vi "Autonomous Independent.vi"() -> ()   [LabVIEW 2023]
doc: "This VI is called when autonomous begins, and will automatically be terminated when autonomous ends. You can carry out timed or sensor driven robot movement independently without needing to return to the caller."
uses:
  <vilib>/Rock Robotics/WPI/ThirdParty/REV Robotics/REVLib/Typedef/Spark MAX Idle Mode.ctl
  <vilib>/Rock Robotics/WPI/SafetyOutput/WPI_SafetyOutputConfigMenu.ctl
  <vilib>/Rock Robotics/Network Tables/NT Read String.vi
  <vilib>/Rock Robotics/WPI/Utilities/WPI_GetSetVariantRefNum.vi
panel:
  out "Sensor Position 8":dbl
  out "Sensor Position 7":dbl
  out "?":dbl
  out "Sensor Position 6":dbl
  out "Sensor Position 5":dbl
  out "Sensor Position 4":dbl
  out "Sensor Position 3":dbl
  out "Sensor Position 2":dbl
  out "Sensor Position":dbl
  out "?":dbl
  # "Autonomous Independent.viBe sure to right-click and choose Data Operations>>Make Current Value default if you want to save the array values with the VI"
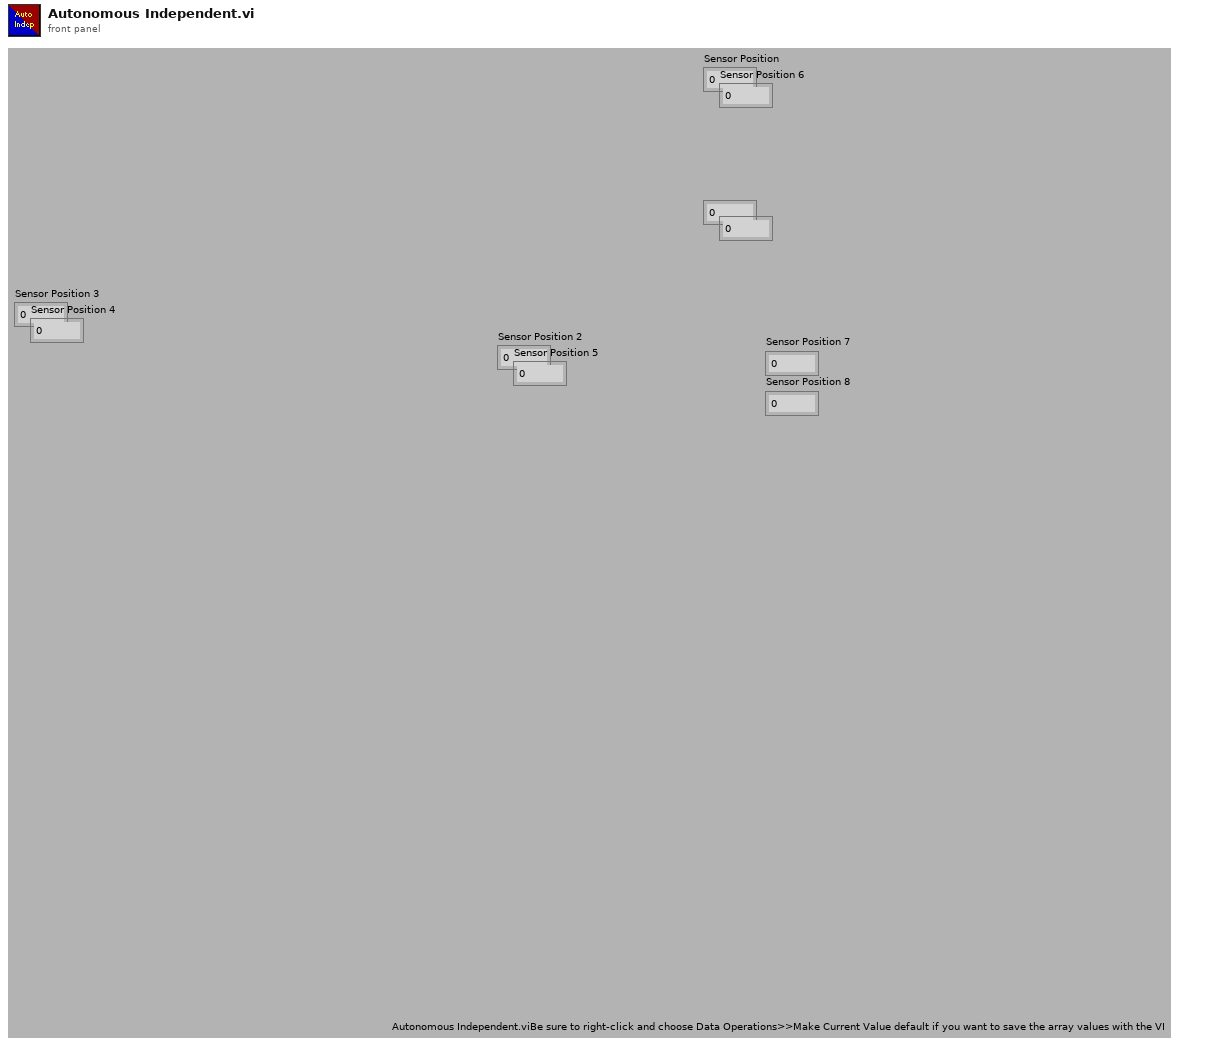
[diagram p1: front panel]
types:
  T1 = typedef "WPI_SafetyOutputConfigMenu.ctl" = enum16{"Enable", "Disable"}
  T2 = enum16{"ação 1", "ação 2", "ação 3", "ação 4", "ação 5", "ação 7", "ação 8"}
  T3 = typedef "Spark MAX Idle Mode.ctl" = enum16{"Coast", "Brake"}
  T4 = enum16{"ação 1", "ação 2", "ação 3", "ação 4", "ação 5"}
  T5 = typedef "WPI_RobotDriveDevRef.ctl" = cluster{"DevStatus":errorcluster, "Motors[]":T6[], "Square Inputs":bool, "Max Output":dbl}
  T6 = typedef "WPI_MotorControlDeviceRef.ctl" = cluster{"DeviceStatus":errorcluster, "Type":T7, "PWM":cluster{"PWM Channel":T8, "DeadBand":T9}, "CAN":cluster{"Device Number":u8, "SetOutput VI Ref":variant, "GetOutput VI Ref":variant, "Enable VI Ref":variant, "Disable VI Ref":variant, "Data":variant}, "Invert":bool, "DIO PWM":cluster{"PWM \"Enable\" Channel":T8, "DIOChannel":T10, "PWM Rate":dbl}}
  T7 = typedef "WPI_MotorControlType.ctl" = enum16{"PWM", "CAN", "DIO PWM"}
  T8 = typedef "FPGA_DIOPWMChannel.ctl" = enum8{"PWM 0", "PWM 1", "PWM 2", "PWM 3", "PWM 4", "PWM 5", "PWM 6", "PWM 7", "PWM 8", "PWM 9", "PWM MXP 0", "PWM MXP 1", "PWM MXP 2", "PWM MXP 3", "PWM MXP 4", "PWM MXP 5", "PWM MXP 6", "PWM MXP 7", "PWM MXP 8", "PWM MXP 9", "Invalid"}
  T9 = typedef "WPI_PWMDeadband.ctl" = cluster{"Name":string, "maxPositivePwm":i32, "minPositivePwm":i32, "centerPwm":i32, "maxNegativePwm":i32, "minNegativePwm":i32, "angularRange":u16}
  T10 = typedef "FPGA_DIOChannel.ctl" = enum8{"DIO 0", "DIO 1", "DIO 2", "DIO 3", "DIO 4", "DIO 5", "DIO 6", "DIO 7", "DIO 8", "DIO 9", "DIO MXP 0", "DIO MXP 1", "DIO MXP 2", "DIO MXP 3", "DIO MXP 4", "DIO MXP 5", "DIO MXP 6", "DIO MXP 7", "DIO MXP 8", "DIO MXP 9", "DIO MXP 10", "DIO MXP 11", "DIO MXP 12", "DIO MXP 13", "DIO MXP 14", "DIO MXP 15", "SPI Port CS1", "SPI Port CS2", "SPI Port CS3", "SPI Port MISO", "SPI Port MOSI", "Invalid"}
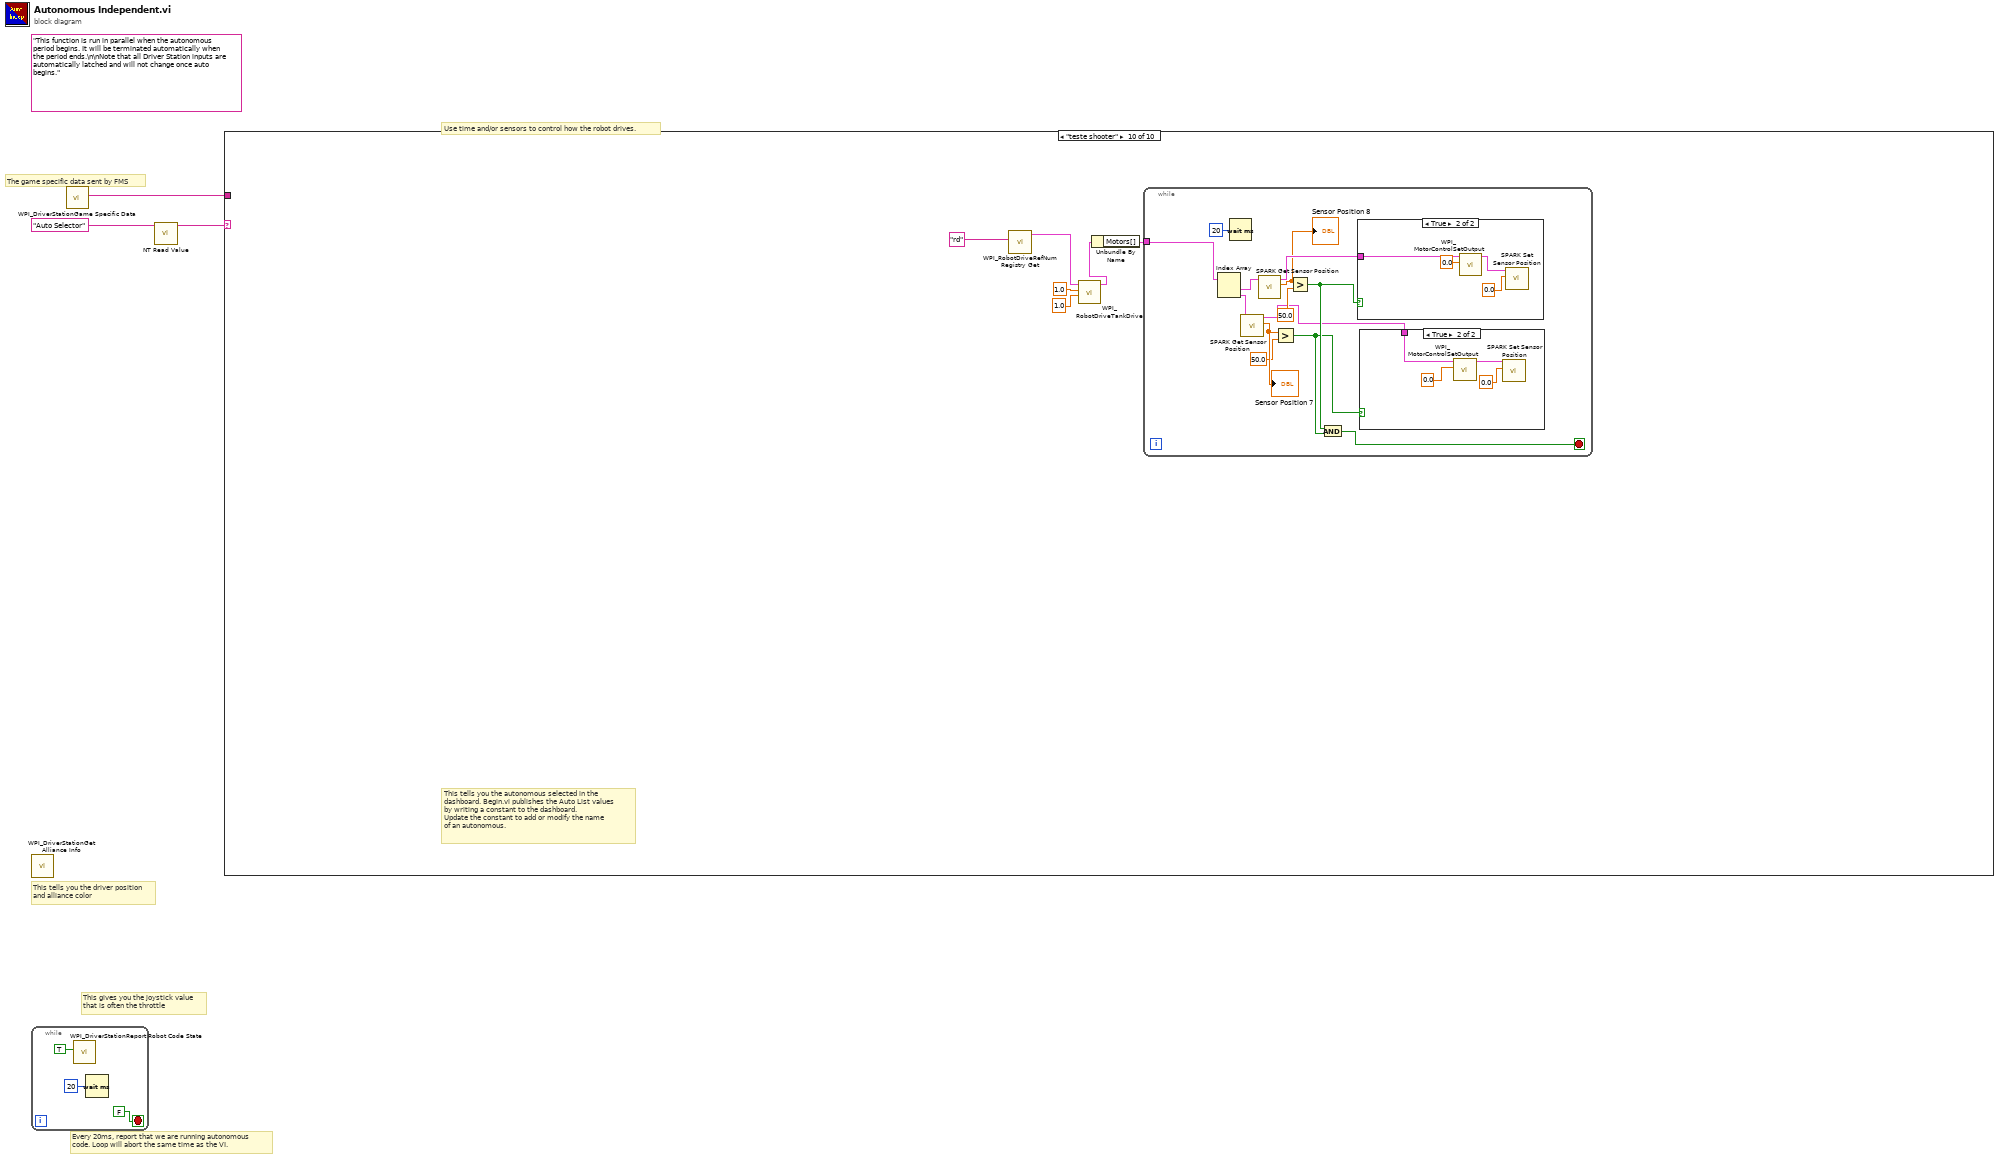
[diagram p0: block diagram]
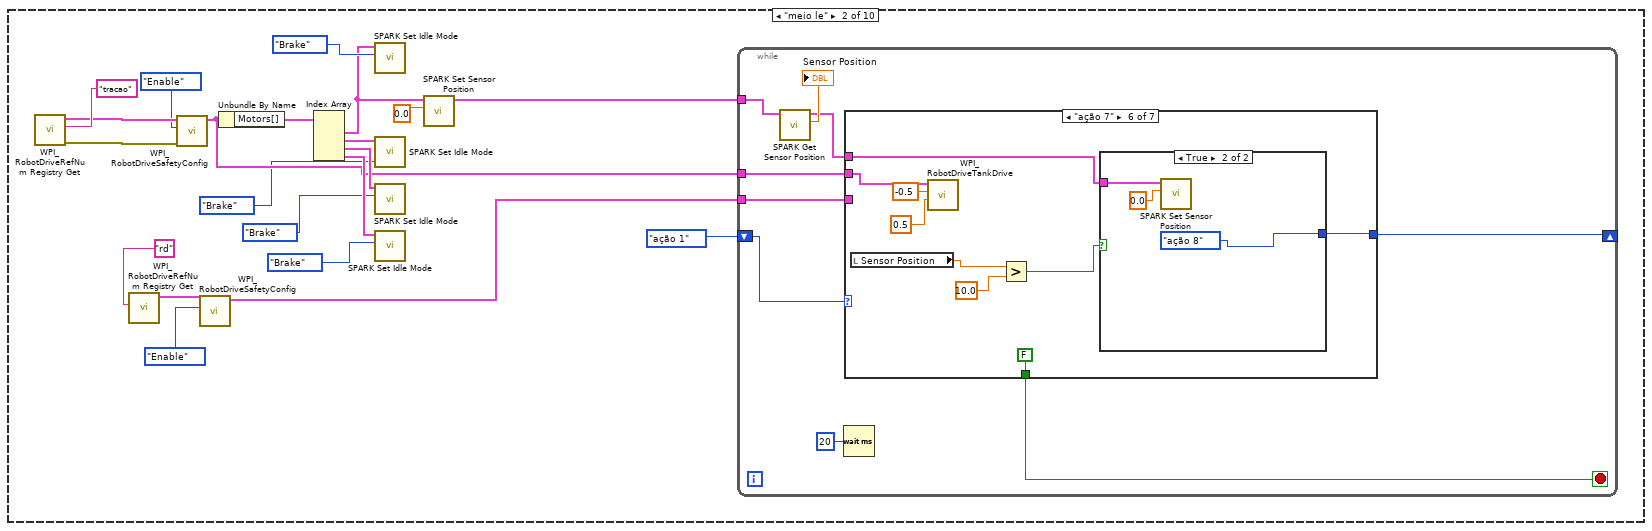
[diagram p3: hidden frame]
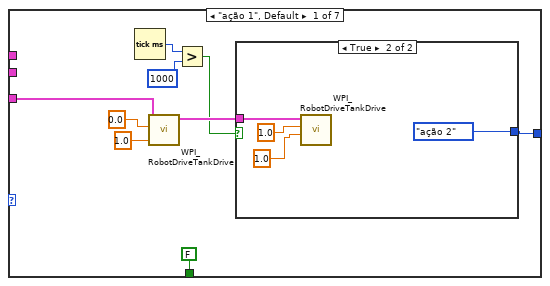
[diagram p4: hidden frame]
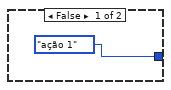
[diagram p5: hidden frame]
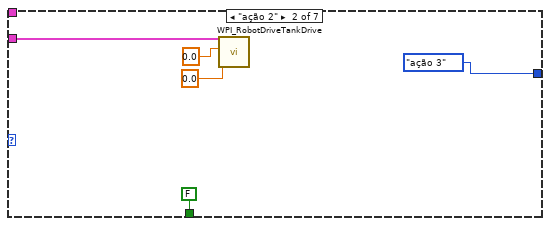
[diagram p6: hidden frame]
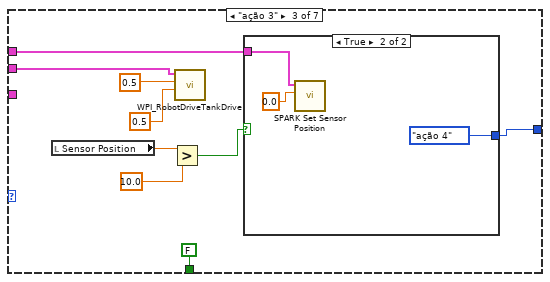
[diagram p7: hidden frame]
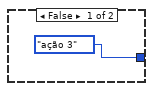
[diagram p8: hidden frame]
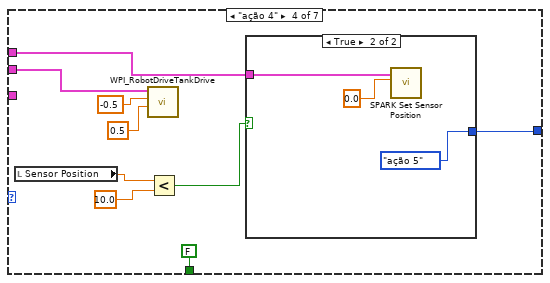
[diagram p9: hidden frame]
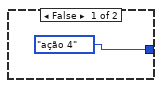
[diagram p10: hidden frame]
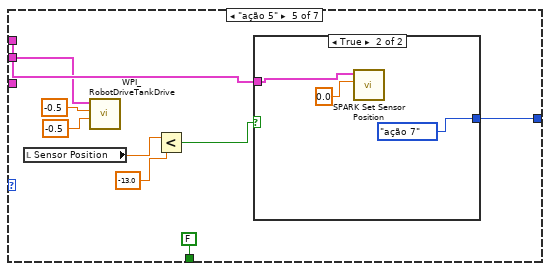
[diagram p11: hidden frame]
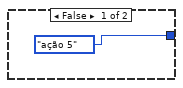
[diagram p12: hidden frame]
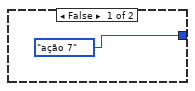
[diagram p13: hidden frame]
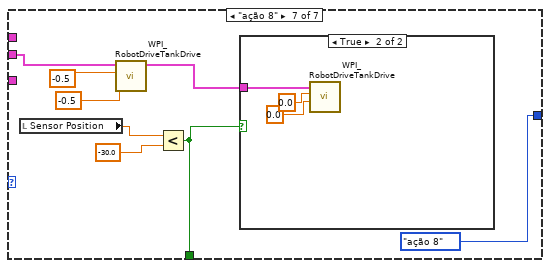
[diagram p14: hidden frame]
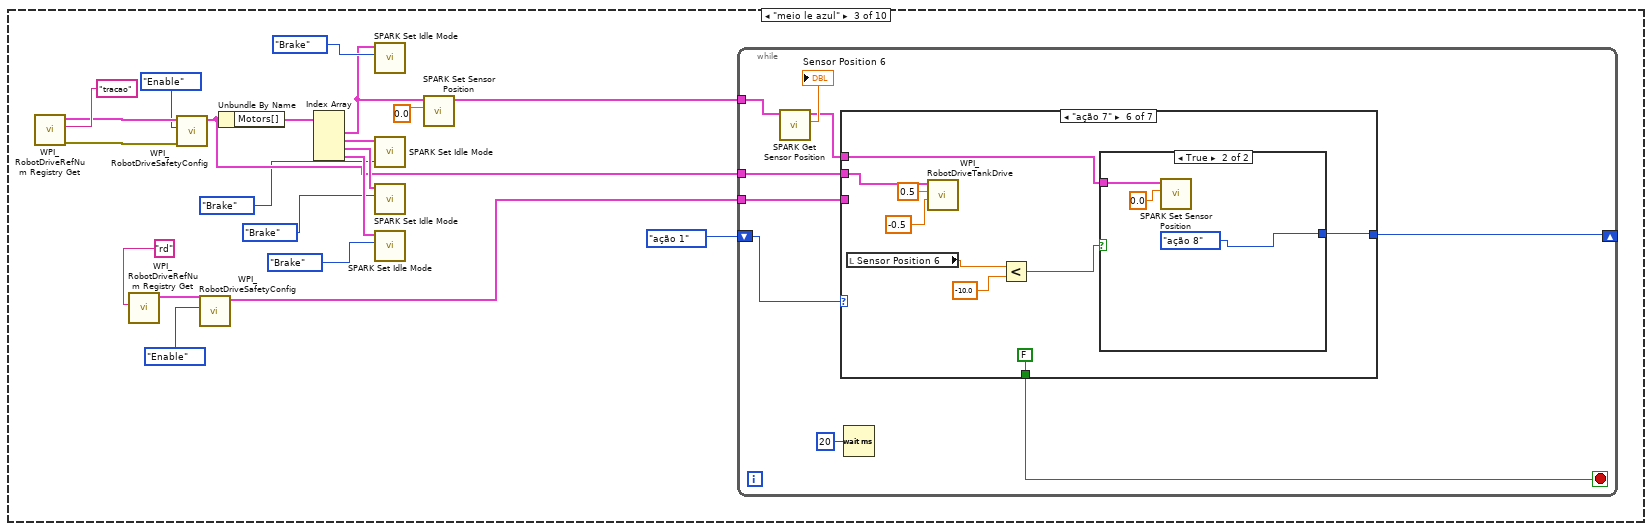
[diagram p16: hidden frame]
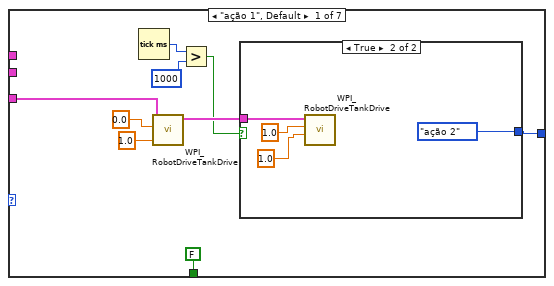
[diagram p17: hidden frame]
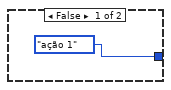
[diagram p18: hidden frame]
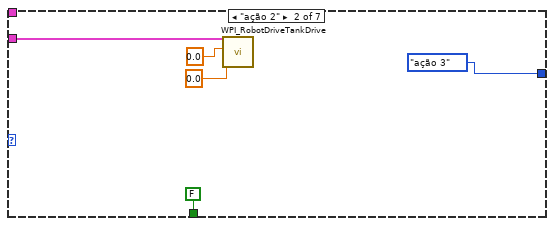
[diagram p19: hidden frame]
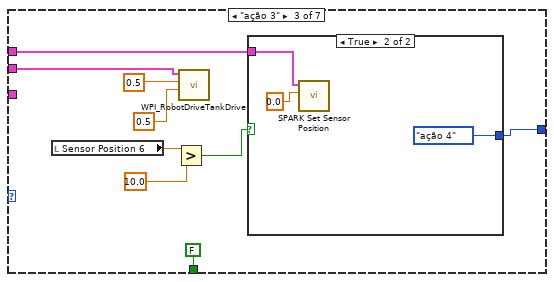
[diagram p20: hidden frame]
diagram:
  (unwired) "This function is run in parallel when the autonomous period begins. It will be terminated automatically when the period ends.\n\nNote that all Driver Station inputs are automatically latched and will not change once auto begins."
  # "The game specific data sent by FMS"
  # "This tells you the autonomous selected in the \ndashboard. Begin.vi publishes the Auto List values\nby writing a constant to the dashboard.\nUpdate the constant to add or modify the name\nof an autonomous."
  # "Every 20ms, report that we are running autonomous\ncode. Loop will abort the same time as the VI."
  # "This gives you the joystick value\nthat is often the throttle"
  # "Use time and/or sensors to control how the robot drives."
  # "This tells you the driver position\nand alliance color"
  n1 = call <vilib>:"WPI_DriverStationGet Alliance Info.vi"() -> ()  [unwired: 12 out]
  n2 = while {
    stop <- FALSE stop-if-true
    n3 = call <vilib>:"WPI_DriverStationReport Robot Code State.vi"("Autonomous"=TRUE) -> ()  [unwired: 10 in, 1 out]
    n4 = Wait (ms)(milliseconds to wait=u32 20) -> ()  [unwired: 1 out]
  }
  n5 = call <vilib>:"WPI_DriverStationGame Specific Data.vi"() -> ("Game Specific Data"=w1:string)  [unwired: 11 in]
  n6 = call-poly <vilib>:"NT Read Value.vi"("name"="Auto Selector" ("Name")) -> ("value"=w2:string)  [unwired: 8 in, 2 out]
  n7 = case shown="\"teste shooter\"" w2 {
    tunnel: w1 -> [_ _ _ _ _ _ _ _ _ _]
    frame Default {
    }
    frame "meio le" {
      n8 = call <vilib>:"WPI_RobotDriveRefNum Registry Get.vi"("refnum name"="tracao") -> ("error out"=w26:errorcluster, "RobotDriveDevRef"=w25:T5)  [unwired: 9 in]
      n9 = call <vilib>:"WPI_RobotDriveRefNum Registry Get.vi"("refnum name"="rd") -> ("RobotDriveDevRef"=w15:T5)  [unwired: 9 in, 1 out]
      n10 = call <vilib>:"WPI_RobotDriveSafetyConfig.vi"("error in (no error)"=w26, "mode"=WPI_SafetyOutputConfigMenu."Enable", "RobotDriveDevRef"=w25) -> ("RobotDriveDevRef"=w13:T5)  [unwired: 7 in, 1 out]
      n11 = call <vilib>:"WPI_RobotDriveSafetyConfig.vi"("mode"=WPI_SafetyOutputConfigMenu."Enable", "RobotDriveDevRef"=w15) -> ("RobotDriveDevRef"=w14:T5)  [unwired: 8 in, 1 out]
      n12 = Unbundle By Name(w13) -> ("Motors[]"=w24:T6[])
      n13 = Index Array(array=w24) -> (element #1=w17:T6, element #2=w21:T6, element #3=w20:T6, element #4=w19:T6)  [unwired: 4 in]
      n14 = call <vilib>:"SPARK Set Idle Mode.vi"("Idle Mode"=Spark_MAX_Idle_Mode."Brake", "MotorControlDeviceRef in"=w17) -> ()  [unwired: 8 in, 2 out]
      n15 = call <vilib>:"SPARK Set Idle Mode.vi"("Idle Mode"=Spark_MAX_Idle_Mode."Brake", "MotorControlDeviceRef in"=w21) -> ()  [unwired: 8 in, 2 out]
      n16 = call <vilib>:"SPARK Set Idle Mode.vi"("Idle Mode"=Spark_MAX_Idle_Mode."Brake", "MotorControlDeviceRef in"=w20) -> ()  [unwired: 8 in, 2 out]
      n17 = call <vilib>:"SPARK Set Idle Mode.vi"("Idle Mode"=Spark_MAX_Idle_Mode."Brake", "MotorControlDeviceRef in"=w19) -> ()  [unwired: 8 in, 2 out]
      n18 = call <vilib>:"SPARK Set Sensor Position.vi"("Position"=0.0, "MotorControlDeviceRef"=w17) -> ("MotorControlDeviceRef"=w12:T6)  [unwired: 8 in, 1 out]
      n19 = while {
        shift-right: [w33] -> _
        shift-left: T2."ação 1" -> [w35]
        tunnel: w14 -> [w34]
        tunnel: w13 -> [w32]
        tunnel: w12 -> [w30]
        stop <- w28 stop-if-true
        n20 = call <vilib>:"SPARK Get Sensor Position.vi"("MotorControlDevRef in"=w30) -> ("Sensor Position"=→"Sensor Position":dbl, "MotorControlDevRef out"=w29:T6)  [unwired: 7 in, 2 out]
        n21 = Wait (ms)(milliseconds to wait=u32 20) -> ()  [unwired: 1 out]
        n22 = case shown="\"ação 7\"" w35 {
          tunnel: w34 -> [w43 w55 _ _ _ _ _]
          tunnel: [w38 T2."ação 3" w57 w70 w83 w96 T2."ação 8"] -> w33
          tunnel: w32 -> [_ _ w64 w77 w87 w103 w115]
          tunnel: w29 -> [_ _ w58 w71 w90 w97 _]
          tunnel: [FALSE FALSE FALSE FALSE FALSE FALSE w109] -> w28
          frame "ação 1", Default {
            n23 = Tick Count (ms)() -> (millisecond timer value=w41:u32)
            n24 = call <vilib>:"WPI_RobotDriveTankDrive.vi"("Right axis value"=1.0, "Left axis value"=0.0, "RobotDriveDevRef"=w43) -> ("RobotDriveDevRef"=w42:T5)  [unwired: 6 in, 2 out]
            n25 = Greater?(x=w41, y=u32 1000) -> (0:w39:bool)
            n26 = case shown="True" w39 {
              tunnel: w42 -> [_ w48]
              tunnel: [T2."ação 1" T2."ação 2"] -> w38
              frame False {
              }
              frame True {
                n27 = call <vilib>:"WPI_RobotDriveTankDrive.vi"("Right axis value"=1.0 ("Left axis value"), "Left axis value"=1.0 ("Right axis value"), "RobotDriveDevRef"=w48) -> ()  [unwired: 6 in, 3 out]
              }
            }
          }
          frame "ação 2" {
            n28 = call <vilib>:"WPI_RobotDriveTankDrive.vi"("Right axis value"=0.0, "Left axis value"=0.0, "RobotDriveDevRef"=w55) -> ()  [unwired: 6 in, 3 out]
          }
          frame "ação 3" {
            n29 = local read "Sensor Position"() -> (w60:dbl)
            n30 = Greater?(x=w60, y=10.0) -> (0:w61:bool)
            n31 = call <vilib>:"WPI_RobotDriveTankDrive.vi"("Right axis value"=0.5 ("Left axis value"), "Left axis value"=0.5, "RobotDriveDevRef"=w64) -> ()  [unwired: 6 in, 3 out]
            n32 = case shown="True" w61 {
              tunnel: w58 -> [_ w68]
              tunnel: [T2."ação 3" T2."ação 4"] -> w57
              frame False {
              }
              frame True {
                n33 = call <vilib>:"SPARK Set Sensor Position.vi"("Position"=0.0, "MotorControlDeviceRef"=w68) -> ()  [unwired: 8 in, 2 out]
              }
            }
          }
          frame "ação 4" {
            n34 = local read "Sensor Position"() -> (w74:dbl)
            n35 = call <vilib>:"WPI_RobotDriveTankDrive.vi"("Right axis value"=0.5 ("Left axis value"), "Left axis value"=-0.5, "RobotDriveDevRef"=w77) -> ()  [unwired: 6 in, 3 out]
            n36 = Less?(x=w74, y=10.0) -> (x < y?=w72:bool)
            n37 = case shown="True" w72 {
              tunnel: w71 -> [_ w81]
              tunnel: [T2."ação 4" T2."ação 5"] -> w70
              frame False {
              }
              frame True {
                n38 = call <vilib>:"SPARK Set Sensor Position.vi"("Position"=0.0, "MotorControlDeviceRef"=w81) -> ()  [unwired: 8 in, 2 out]
              }
            }
          }
          frame "ação 5" {
            n39 = local read "Sensor Position"() -> (w86:dbl)
            n40 = call <vilib>:"WPI_RobotDriveTankDrive.vi"("Right axis value"=-0.5 ("Left axis value"), "Left axis value"=-0.5, "RobotDriveDevRef"=w87) -> ()  [unwired: 6 in, 3 out]
            n41 = Less?(x=w86, y=-13.0) -> (x < y?=w84:bool)
            n42 = case shown="True" w84 {
              tunnel: w90 -> [_ w93]
              tunnel: [T2."ação 5" T2."ação 7"] -> w83
              frame False {
              }
              frame True {
                n43 = call <vilib>:"SPARK Set Sensor Position.vi"("Position"=0.0, "MotorControlDeviceRef"=w93) -> ()  [unwired: 8 in, 2 out]
              }
            }
          }
          frame "ação 7" {
            n44 = local read "Sensor Position"() -> (w100:dbl)
            n45 = call <vilib>:"WPI_RobotDriveTankDrive.vi"("Right axis value"=0.5 ("Left axis value"), "Left axis value"=-0.5, "RobotDriveDevRef"=w103) -> ()  [unwired: 6 in, 3 out]
            n46 = Greater?(x=w100, y=10.0) -> (0:w98:bool)
            n47 = case shown="True" w98 {
              tunnel: w97 -> [_ w107]
              tunnel: [T2."ação 7" T2."ação 8"] -> w96
              frame False {
              }
              frame True {
                n48 = call <vilib>:"SPARK Set Sensor Position.vi"("Position"=0.0, "MotorControlDeviceRef"=w107) -> ()  [unwired: 8 in, 2 out]
              }
            }
          }
          frame "ação 8" {
            n49 = local read "Sensor Position"() -> (w112:dbl)
            n50 = call <vilib>:"WPI_RobotDriveTankDrive.vi"("Right axis value"=-0.5 ("Left axis value"), "Left axis value"=-0.5, "RobotDriveDevRef"=w115) -> ("RobotDriveDevRef"=w110:T5)  [unwired: 6 in, 2 out]
            n51 = Less?(x=w112, y=-30.0) -> (x < y?=w109:bool)
            n52 = case shown="True" w109 {
              tunnel: w110 -> [_ w118]
              frame False {
              }
              frame True {
                n53 = call <vilib>:"WPI_RobotDriveTankDrive.vi"("Right axis value"=0.0 ("Left axis value"), "Left axis value"=0.0, "RobotDriveDevRef"=w118) -> ()  [unwired: 6 in, 3 out]
              }
            }
          }
        }
      }
    }
    frame "meio le azul" {
      n54 = call <vilib>:"WPI_RobotDriveRefNum Registry Get.vi"("refnum name"="tracao") -> ("error out"=w138:errorcluster, "RobotDriveDevRef"=w137:T5)  [unwired: 9 in]
      n55 = call <vilib>:"WPI_RobotDriveRefNum Registry Get.vi"("refnum name"="rd") -> ("RobotDriveDevRef"=w127:T5)  [unwired: 9 in, 1 out]
      n56 = call <vilib>:"WPI_RobotDriveSafetyConfig.vi"("error in (no error)"=w138, "mode"=WPI_SafetyOutputConfigMenu."Enable", "RobotDriveDevRef"=w137) -> ("RobotDriveDevRef"=w125:T5)  [unwired: 7 in, 1 out]
      n57 = call <vilib>:"WPI_RobotDriveSafetyConfig.vi"("mode"=WPI_SafetyOutputConfigMenu."Enable", "RobotDriveDevRef"=w127) -> ("RobotDriveDevRef"=w126:T5)  [unwired: 8 in, 1 out]
      n58 = Unbundle By Name(w125) -> ("Motors[]"=w136:T6[])
      n59 = Index Array(array=w136) -> (element #1=w129:T6, element #2=w133:T6, element #3=w132:T6, element #4=w131:T6)  [unwired: 4 in]
      n60 = call <vilib>:"SPARK Set Idle Mode.vi"("Idle Mode"=Spark_MAX_Idle_Mode."Brake", "MotorControlDeviceRef in"=w129) -> ()  [unwired: 8 in, 2 out]
      n61 = call <vilib>:"SPARK Set Idle Mode.vi"("Idle Mode"=Spark_MAX_Idle_Mode."Brake", "MotorControlDeviceRef in"=w133) -> ()  [unwired: 8 in, 2 out]
      n62 = call <vilib>:"SPARK Set Idle Mode.vi"("Idle Mode"=Spark_MAX_Idle_Mode."Brake", "MotorControlDeviceRef in"=w132) -> ()  [unwired: 8 in, 2 out]
      n63 = call <vilib>:"SPARK Set Idle Mode.vi"("Idle Mode"=Spark_MAX_Idle_Mode."Brake", "MotorControlDeviceRef in"=w131) -> ()  [unwired: 8 in, 2 out]
      n64 = call <vilib>:"SPARK Set Sensor Position.vi"("Position"=0.0, "MotorControlDeviceRef"=w129) -> ("MotorControlDeviceRef"=w124:T6)  [unwired: 8 in, 1 out]
      n65 = while {
        shift-right: [w145] -> _
        shift-left: T2."ação 1" -> [w147]
        tunnel: w126 -> [w146]
        tunnel: w125 -> [w144]
        tunnel: w124 -> [w142]
        stop <- w140 stop-if-true
        n66 = call <vilib>:"SPARK Get Sensor Position.vi"("MotorControlDevRef in"=w142) -> ("Sensor Position"=→"Sensor Position 6":dbl, "MotorControlDevRef out"=w141:T6)  [unwired: 7 in, 2 out]
        n67 = case shown="\"ação 7\"" w147 {
          tunnel: w146 -> [w155 w167 _ _ _ _ _]
          tunnel: [w150 T2."ação 3" w169 w182 w195 w208 T2."ação 8"] -> w145
          tunnel: w144 -> [_ _ w176 w189 w199 w215 w227]
          tunnel: w141 -> [_ _ w170 w183 w202 w209 _]
          tunnel: [FALSE FALSE FALSE FALSE FALSE FALSE w221] -> w140
          frame "ação 1", Default {
            n68 = Tick Count (ms)() -> (millisecond timer value=w153:u32)
            n69 = call <vilib>:"WPI_RobotDriveTankDrive.vi"("Right axis value"=1.0, "Left axis value"=0.0, "RobotDriveDevRef"=w155) -> ("RobotDriveDevRef"=w154:T5)  [unwired: 6 in, 2 out]
            n70 = Greater?(x=w153, y=u32 1000) -> (0:w151:bool)
            n71 = case shown="True" w151 {
              tunnel: w154 -> [_ w160]
              tunnel: [T2."ação 1" T2."ação 2"] -> w150
              frame False {
              }
              frame True {
                n72 = call <vilib>:"WPI_RobotDriveTankDrive.vi"("Right axis value"=1.0 ("Left axis value"), "Left axis value"=1.0 ("Right axis value"), "RobotDriveDevRef"=w160) -> ()  [unwired: 6 in, 3 out]
              }
            }
          }
          frame "ação 2" {
            n73 = call <vilib>:"WPI_RobotDriveTankDrive.vi"("Right axis value"=0.0, "Left axis value"=0.0, "RobotDriveDevRef"=w167) -> ()  [unwired: 6 in, 3 out]
          }
          frame "ação 3" {
            n74 = local read "Sensor Position 6"() -> (w172:dbl)
            n75 = Greater?(x=w172, y=10.0) -> (0:w173:bool)
            n76 = call <vilib>:"WPI_RobotDriveTankDrive.vi"("Right axis value"=0.5 ("Left axis value"), "Left axis value"=0.5, "RobotDriveDevRef"=w176) -> ()  [unwired: 6 in, 3 out]
            n77 = case shown="True" w173 {
              tunnel: w170 -> [_ w180]
              tunnel: [T2."ação 3" T2."ação 4"] -> w169
              frame False {
              }
              frame True {
                n78 = call <vilib>:"SPARK Set Sensor Position.vi"("Position"=0.0, "MotorControlDeviceRef"=w180) -> ()  [unwired: 8 in, 2 out]
              }
            }
          }
          frame "ação 4" {
            n79 = local read "Sensor Position 6"() -> (w186:dbl)
            n80 = call <vilib>:"WPI_RobotDriveTankDrive.vi"("Right axis value"=-0.5 ("Left axis value"), "Left axis value"=0.5, "RobotDriveDevRef"=w189) -> ()  [unwired: 6 in, 3 out]
            n81 = Less?(x=w186, y=-10.0) -> (x < y?=w184:bool)
            n82 = case shown="True" w184 {
              tunnel: w183 -> [_ w193]
              tunnel: [T2."ação 4" T2."ação 5"] -> w182
              frame False {
              }
              frame True {
                n83 = call <vilib>:"SPARK Set Sensor Position.vi"("Position"=0.0, "MotorControlDeviceRef"=w193) -> ()  [unwired: 8 in, 2 out]
              }
            }
          }
          frame "ação 5" {
            n84 = local read "Sensor Position 6"() -> (w198:dbl)
            n85 = call <vilib>:"WPI_RobotDriveTankDrive.vi"("Right axis value"=-0.5 ("Left axis value"), "Left axis value"=-0.5, "RobotDriveDevRef"=w199) -> ()  [unwired: 6 in, 3 out]
            n86 = Less?(x=w198, y=-13.0) -> (x < y?=w196:bool)
            n87 = case shown="True" w196 {
              tunnel: w202 -> [_ w205]
              tunnel: [T2."ação 5" T2."ação 7"] -> w195
              frame False {
              }
              frame True {
                n88 = call <vilib>:"SPARK Set Sensor Position.vi"("Position"=0.0, "MotorControlDeviceRef"=w205) -> ()  [unwired: 8 in, 2 out]
              }
            }
          }
          frame "ação 7" {
            n89 = local read "Sensor Position 6"() -> (w212:dbl)
            n90 = call <vilib>:"WPI_RobotDriveTankDrive.vi"("Right axis value"=-0.5 ("Left axis value"), "Left axis value"=0.5, "RobotDriveDevRef"=w215) -> ()  [unwired: 6 in, 3 out]
            n91 = Less?(x=w212, y=-10.0) -> (x < y?=w210:bool)
            n92 = case shown="True" w210 {
              tunnel: w209 -> [_ w219]
              tunnel: [T2."ação 7" T2."ação 8"] -> w208
              frame False {
              }
              frame True {
                n93 = call <vilib>:"SPARK Set Sensor Position.vi"("Position"=0.0, "MotorControlDeviceRef"=w219) -> ()  [unwired: 8 in, 2 out]
              }
            }
          }
          frame "ação 8" {
            n94 = local read "Sensor Position 6"() -> (w224:dbl)
            n95 = call <vilib>:"WPI_RobotDriveTankDrive.vi"("Right axis value"=-0.5 ("Left axis value"), "Left axis value"=-0.5, "RobotDriveDevRef"=w227) -> ("RobotDriveDevRef"=w222:T5)  [unwired: 6 in, 2 out]
            n96 = Less?(x=w224, y=-30.0) -> (x < y?=w221:bool)
            n97 = case shown="True" w221 {
              tunnel: w222 -> [_ w230]
              frame False {
              }
              frame True {
                n98 = call <vilib>:"WPI_RobotDriveTankDrive.vi"("Right axis value"=0.0 ("Left axis value"), "Left axis value"=0.0, "RobotDriveDevRef"=w230) -> ()  [unwired: 6 in, 3 out]
              }
            }
          }
        }
        n99 = Wait (ms)(milliseconds to wait=u32 20) -> ()  [unwired: 1 out]
      }
    }
    frame "direita" {
      n100 = call <vilib>:"WPI_RobotDriveRefNum Registry Get.vi"("refnum name"="rd") -> ("RobotDriveDevRef"=w233:T5)  [unwired: 9 in, 1 out]
      n101 = call <vilib>:"WPI_RobotDriveRefNum Registry Get.vi"("refnum name"="tracao") -> ("error out"=w250:errorcluster, "RobotDriveDevRef"=w249:T5)  [unwired: 9 in]
      n102 = call <vilib>:"WPI_RobotDriveSafetyConfig.vi"("mode"=WPI_SafetyOutputConfigMenu."Enable", "RobotDriveDevRef"=w233) -> ("RobotDriveDevRef"=w232:T5)  [unwired: 8 in, 1 out]
      n103 = call <vilib>:"WPI_RobotDriveSafetyConfig.vi"("error in (no error)"=w250, "mode"=WPI_SafetyOutputConfigMenu."Enable", "RobotDriveDevRef"=w249) -> ("RobotDriveDevRef"=w235:T5)  [unwired: 7 in, 1 out]
      n104 = Unbundle By Name(w235) -> ("Motors[]"=w247:T6[])
      n105 = Index Array(array=w247) -> (element #1=w239:T6, element #2=w242:T6, element #3=w241:T6, element #4=w240:T6)  [unwired: 4 in]
      n106 = call <vilib>:"SPARK Set Idle Mode.vi"("Idle Mode"=Spark_MAX_Idle_Mode."Brake", "MotorControlDeviceRef in"=w239) -> ()  [unwired: 8 in, 2 out]
      n107 = call <vilib>:"SPARK Set Idle Mode.vi"("Idle Mode"=Spark_MAX_Idle_Mode."Brake", "MotorControlDeviceRef in"=w242) -> ()  [unwired: 8 in, 2 out]
      n108 = call <vilib>:"SPARK Set Idle Mode.vi"("Idle Mode"=Spark_MAX_Idle_Mode."Brake", "MotorControlDeviceRef in"=w241) -> ()  [unwired: 8 in, 2 out]
      n109 = call <vilib>:"SPARK Set Idle Mode.vi"("Idle Mode"=Spark_MAX_Idle_Mode."Brake", "MotorControlDeviceRef in"=w240) -> ()  [unwired: 8 in, 2 out]
      n110 = call <vilib>:"SPARK Set Sensor Position.vi"("Position"=0.0, "MotorControlDeviceRef"=w239) -> ("MotorControlDeviceRef"=w237:T6)  [unwired: 8 in, 1 out]
      n111 = while {
        shift-right: [w253] -> _
        shift-left: T4."ação 1" -> [w258]
        tunnel: w237 -> [w256]
        tunnel: w235 -> [w254]
        tunnel: w232 -> [w252]
        stop <- w257 stop-if-true
        n112 = call <vilib>:"SPARK Get Sensor Position.vi"("MotorControlDevRef in"=w256) -> ("Sensor Position"=→"?":dbl)  [unwired: 7 in, 3 out]
        n113 = case shown="\"ação 1\", Default" w258 {
          tunnel: [FALSE FALSE FALSE FALSE w304] -> w257
          tunnel: [w261 T4."ação 3" w279 w290 T4."ação 5"] -> w253
          tunnel: w254 -> [_ _ w281 w292 w301]
          tunnel: w252 -> [w260 w274 _ _ _]
          frame "ação 1", Default {
            n114 = Tick Count (ms)() -> (millisecond timer value=w265:u32)
            n115 = call <vilib>:"WPI_RobotDriveTankDrive.vi"("Right axis value"=1.0, "Left axis value"=0.0, "RobotDriveDevRef"=w260) -> ("RobotDriveDevRef"=w266:T5)  [unwired: 6 in, 2 out]
            n116 = Greater?(x=w265, y=u32 1000) -> (0:w263:bool)
            n117 = case shown="True" w263 {
              tunnel: w266 -> [_ w271]
              tunnel: [T4."ação 1" T4."ação 2"] -> w261
              frame False {
              }
              frame True {
                n118 = call <vilib>:"WPI_RobotDriveTankDrive.vi"("Right axis value"=1.0 ("Left axis value"), "Left axis value"=1.0 ("Right axis value"), "RobotDriveDevRef"=w271) -> ()  [unwired: 6 in, 3 out]
              }
            }
          }
          frame "ação 2" {
            n119 = call <vilib>:"WPI_RobotDriveTankDrive.vi"("Right axis value"=0.0 ("Left axis value"), "Left axis value"=0.0, "RobotDriveDevRef"=w274) -> ()  [unwired: 6 in, 3 out]
          }
          frame "ação 3" {
            n120 = local read item#?() -> (w280:dbl)
            n121 = Greater?(x=w280, y=18.5) -> (0:w284:bool)
            n122 = call <vilib>:"WPI_RobotDriveTankDrive.vi"("Right axis value"=0.5 ("Left axis value"), "Left axis value"=0.5, "RobotDriveDevRef"=w281) -> ()  [unwired: 6 in, 3 out]
            n123 = case shown="True" w284 {
              tunnel: [T4."ação 3" T4."ação 4"] -> w279
              frame False {
              }
              frame True {
                n124 = call <vilib>:"SPARK Set Sensor Position.vi"("Position"=0.0) -> ()  [unwired: 9 in, 2 out]
              }
            }
          }
          frame "ação 4" {
            n125 = local read item#?() -> (w291:dbl)
            n126 = call <vilib>:"WPI_RobotDriveTankDrive.vi"("Right axis value"=0.5 ("Left axis value"), "Left axis value"=-0.5, "RobotDriveDevRef"=w292) -> ()  [unwired: 6 in, 3 out]
            n127 = Greater?(x=w291, y=8.5) -> (0:w294:bool)
            n128 = case shown="True" w294 {
              tunnel: [T4."ação 5" T4."ação 5"] -> w290
              frame False {
              }
              frame True {
                n129 = call <vilib>:"SPARK Set Sensor Position.vi"("Position"=0.0) -> ()  [unwired: 9 in, 2 out]
              }
            }
          }
          frame "ação 5" {
            n130 = local read item#?() -> (w303:dbl)
            n131 = call <vilib>:"WPI_RobotDriveTankDrive.vi"("Right axis value"=-0.5 ("Left axis value"), "Left axis value"=-0.5, "RobotDriveDevRef"=w301) -> ("RobotDriveDevRef"=w305:T5)  [unwired: 6 in, 2 out]
            n132 = Less?(x=w303, y=-13.0) -> (x < y?=w304:bool)
            n133 = case shown="True" w304 {
              tunnel: w305 -> [_ w309]
              frame False {
              }
              frame True {
                n134 = call <vilib>:"WPI_RobotDriveTankDrive.vi"("Right axis value"=0.0 ("Left axis value"), "Left axis value"=0.0, "RobotDriveDevRef"=w309) -> ()  [unwired: 6 in, 3 out]
              }
            }
          }
        }
        n135 = Wait (ms)(milliseconds to wait=u32 20) -> ()  [unwired: 1 out]
      }
    }
    frame "direita azul" {
      n136 = call <vilib>:"WPI_RobotDriveRefNum Registry Get.vi"("refnum name"="rd") -> ("RobotDriveDevRef"=w314:T5)  [unwired: 9 in, 1 out]
      n137 = call <vilib>:"WPI_RobotDriveRefNum Registry Get.vi"("refnum name"="tracao") -> ("error out"=w331:errorcluster, "RobotDriveDevRef"=w330:T5)  [unwired: 9 in]
      n138 = call <vilib>:"WPI_RobotDriveSafetyConfig.vi"("mode"=WPI_SafetyOutputConfigMenu."Enable", "RobotDriveDevRef"=w314) -> ("RobotDriveDevRef"=w313:T5)  [unwired: 8 in, 1 out]
      n139 = call <vilib>:"WPI_RobotDriveSafetyConfig.vi"("error in (no error)"=w331, "mode"=WPI_SafetyOutputConfigMenu."Enable", "RobotDriveDevRef"=w330) -> ("RobotDriveDevRef"=w316:T5)  [unwired: 7 in, 1 out]
      n140 = Unbundle By Name(w316) -> ("Motors[]"=w328:T6[])
      n141 = Index Array(array=w328) -> (element #1=w320:T6, element #2=w323:T6, element #3=w322:T6, element #4=w321:T6)  [unwired: 4 in]
      n142 = call <vilib>:"SPARK Set Idle Mode.vi"("Idle Mode"=Spark_MAX_Idle_Mode."Brake", "MotorControlDeviceRef in"=w320) -> ()  [unwired: 8 in, 2 out]
      n143 = call <vilib>:"SPARK Set Idle Mode.vi"("Idle Mode"=Spark_MAX_Idle_Mode."Brake", "MotorControlDeviceRef in"=w323) -> ()  [unwired: 8 in, 2 out]
      n144 = call <vilib>:"SPARK Set Idle Mode.vi"("Idle Mode"=Spark_MAX_Idle_Mode."Brake", "MotorControlDeviceRef in"=w322) -> ()  [unwired: 8 in, 2 out]
      n145 = call <vilib>:"SPARK Set Idle Mode.vi"("Idle Mode"=Spark_MAX_Idle_Mode."Brake", "MotorControlDeviceRef in"=w321) -> ()  [unwired: 8 in, 2 out]
      n146 = call <vilib>:"SPARK Set Sensor Position.vi"("Position"=0.0, "MotorControlDeviceRef"=w320) -> ("MotorControlDeviceRef"=w318:T6)  [unwired: 8 in, 1 out]
      n147 = while {
        shift-right: [w334] -> _
        shift-left: T4."ação 1" -> [w339]
        tunnel: w318 -> [w337]
        tunnel: w316 -> [w335]
        tunnel: w313 -> [w333]
        stop <- w338 stop-if-true
        n148 = call <vilib>:"SPARK Get Sensor Position.vi"("MotorControlDevRef in"=w337) -> ("Sensor Position"=→"?":dbl)  [unwired: 7 in, 3 out]
        n149 = case shown="\"ação 5\"" w339 {
          tunnel: [FALSE FALSE FALSE FALSE w385] -> w338
          tunnel: [w342 T4."ação 3" w360 w371 T4."ação 5"] -> w334
          tunnel: w335 -> [_ _ w362 w373 w382]
          tunnel: w333 -> [w341 w355 _ _ _]
          frame "ação 1", Default {
            n150 = Tick Count (ms)() -> (millisecond timer value=w346:u32)
            n151 = call <vilib>:"WPI_RobotDriveTankDrive.vi"("Right axis value"=1.0, "Left axis value"=0.0, "RobotDriveDevRef"=w341) -> ("RobotDriveDevRef"=w347:T5)  [unwired: 6 in, 2 out]
            n152 = Greater?(x=w346, y=u32 1000) -> (0:w344:bool)
            n153 = case shown="True" w344 {
              tunnel: w347 -> [_ w352]
              tunnel: [T4."ação 1" T4."ação 2"] -> w342
              frame False {
              }
              frame True {
                n154 = call <vilib>:"WPI_RobotDriveTankDrive.vi"("Right axis value"=1.0 ("Left axis value"), "Left axis value"=1.0 ("Right axis value"), "RobotDriveDevRef"=w352) -> ()  [unwired: 6 in, 3 out]
              }
            }
          }
          frame "ação 2" {
            n155 = call <vilib>:"WPI_RobotDriveTankDrive.vi"("Right axis value"=0.0 ("Left axis value"), "Left axis value"=0.0, "RobotDriveDevRef"=w355) -> ()  [unwired: 6 in, 3 out]
          }
          frame "ação 3" {
            n156 = local read item#7() -> (w361:dbl)
            n157 = Greater?(x=w361, y=18.5) -> (0:w365:bool)
            n158 = call <vilib>:"WPI_RobotDriveTankDrive.vi"("Right axis value"=0.5 ("Left axis value"), "Left axis value"=0.5, "RobotDriveDevRef"=w362) -> ()  [unwired: 6 in, 3 out]
            n159 = case shown="True" w365 {
              tunnel: [T4."ação 3" T4."ação 4"] -> w360
              frame False {
              }
              frame True {
                n160 = call <vilib>:"SPARK Set Sensor Position.vi"("Position"=0.0) -> ()  [unwired: 9 in, 2 out]
              }
            }
          }
          frame "ação 4" {
            n161 = local read item#7() -> (w372:dbl)
            n162 = call <vilib>:"WPI_RobotDriveTankDrive.vi"("Right axis value"=-0.5 ("Left axis value"), "Left axis value"=0.5, "RobotDriveDevRef"=w373) -> ()  [unwired: 6 in, 3 out]
            n163 = Less?(x=w372, y=-8.5) -> (x < y?=w375:bool)
            n164 = case shown="True" w375 {
              tunnel: [T4."ação 5" T4."ação 5"] -> w371
              frame False {
              }
              frame True {
                n165 = call <vilib>:"SPARK Set Sensor Position.vi"("Position"=0.0) -> ()  [unwired: 9 in, 2 out]
              }
            }
          }
          frame "ação 5" {
            n166 = local read item#7() -> (w384:dbl)
            n167 = call <vilib>:"WPI_RobotDriveTankDrive.vi"("Right axis value"=-0.5 ("Left axis value"), "Left axis value"=-0.5, "RobotDriveDevRef"=w382) -> ("RobotDriveDevRef"=w386:T5)  [unwired: 6 in, 2 out]
            n168 = Less?(x=w384, y=-13.0) -> (x < y?=w385:bool)
            n169 = case shown="True" w385 {
              tunnel: w386 -> [_ w390]
              frame False {
              }
              frame True {
                n170 = call <vilib>:"WPI_RobotDriveTankDrive.vi"("Right axis value"=0.0 ("Left axis value"), "Left axis value"=0.0, "RobotDriveDevRef"=w390) -> ()  [unwired: 6 in, 3 out]
              }
            }
          }
        }
        n171 = Wait (ms)(milliseconds to wait=u32 20) -> ()  [unwired: 1 out]
      }
    }
    frame "meio ld" {
      n172 = call <vilib>:"WPI_RobotDriveRefNum Registry Get.vi"("refnum name"="tracao") -> ("error out"=w412:errorcluster, "RobotDriveDevRef"=w411:T5)  [unwired: 9 in]
      n173 = call <vilib>:"WPI_RobotDriveRefNum Registry Get.vi"("refnum name"="rd") -> ("RobotDriveDevRef"=w401:T5)  [unwired: 9 in, 1 out]
      n174 = call <vilib>:"WPI_RobotDriveSafetyConfig.vi"("error in (no error)"=w412, "mode"=WPI_SafetyOutputConfigMenu."Enable", "RobotDriveDevRef"=w411) -> ("RobotDriveDevRef"=w399:T5)  [unwired: 7 in, 1 out]
      n175 = call <vilib>:"WPI_RobotDriveSafetyConfig.vi"("mode"=WPI_SafetyOutputConfigMenu."Enable", "RobotDriveDevRef"=w401) -> ("RobotDriveDevRef"=w400:T5)  [unwired: 8 in, 1 out]
      n176 = Unbundle By Name(w399) -> ("Motors[]"=w410:T6[])
      n177 = Index Array(array=w410) -> (element #1=w403:T6, element #2=w407:T6, element #3=w406:T6, element #4=w405:T6)  [unwired: 4 in]
      n178 = call <vilib>:"SPARK Set Idle Mode.vi"("Idle Mode"=Spark_MAX_Idle_Mode."Brake", "MotorControlDeviceRef in"=w403) -> ()  [unwired: 8 in, 2 out]
      n179 = call <vilib>:"SPARK Set Idle Mode.vi"("Idle Mode"=Spark_MAX_Idle_Mode."Brake", "MotorControlDeviceRef in"=w407) -> ()  [unwired: 8 in, 2 out]
      n180 = call <vilib>:"SPARK Set Idle Mode.vi"("Idle Mode"=Spark_MAX_Idle_Mode."Brake", "MotorControlDeviceRef in"=w406) -> ()  [unwired: 8 in, 2 out]
      n181 = call <vilib>:"SPARK Set Idle Mode.vi"("Idle Mode"=Spark_MAX_Idle_Mode."Brake", "MotorControlDeviceRef in"=w405) -> ()  [unwired: 8 in, 2 out]
      n182 = call <vilib>:"SPARK Set Sensor Position.vi"("Position"=0.0, "MotorControlDeviceRef"=w403) -> ("MotorControlDeviceRef"=w398:T6)  [unwired: 8 in, 1 out]
      n183 = while {
        shift-right: [w419] -> _
        shift-left: T2."ação 8" -> [w421]
        tunnel: w400 -> [w420]
        tunnel: w399 -> [w418]
        tunnel: w398 -> [w416]
        stop <- w414 stop-if-true
        n184 = call <vilib>:"SPARK Get Sensor Position.vi"("MotorControlDevRef in"=w416) -> ("Sensor Position"=→"Sensor Position 2":dbl, "MotorControlDevRef out"=w415:T6)  [unwired: 7 in, 2 out]
        n185 = case shown="\"ação 7\"" w421 {
          tunnel: w420 -> [w429 w441 _ _ _ _ _]
          tunnel: [w424 T2."ação 3" w443 w456 w469 w482 T2."ação 8"] -> w419
          tunnel: w418 -> [_ _ w450 w463 w473 w489 w501]
          tunnel: w415 -> [_ _ w444 w457 w476 w483 _]
          tunnel: [FALSE FALSE FALSE FALSE FALSE FALSE w495] -> w414
          frame "ação 1", Default {
            n186 = Tick Count (ms)() -> (millisecond timer value=w427:u32)
            n187 = call <vilib>:"WPI_RobotDriveTankDrive.vi"("Right axis value"=1.0, "Left axis value"=0.0, "RobotDriveDevRef"=w429) -> ("RobotDriveDevRef"=w428:T5)  [unwired: 6 in, 2 out]
            n188 = Greater?(x=w427, y=u32 1000) -> (0:w425:bool)
            n189 = case shown="True" w425 {
              tunnel: w428 -> [_ w434]
              tunnel: [T2."ação 1" T2."ação 2"] -> w424
              frame False {
              }
              frame True {
                n190 = call <vilib>:"WPI_RobotDriveTankDrive.vi"("Right axis value"=1.0 ("Left axis value"), "Left axis value"=1.0 ("Right axis value"), "RobotDriveDevRef"=w434) -> ()  [unwired: 6 in, 3 out]
              }
            }
          }
          frame "ação 2" {
            n191 = call <vilib>:"WPI_RobotDriveTankDrive.vi"("Right axis value"=0.0, "Left axis value"=0.0, "RobotDriveDevRef"=w441) -> ()  [unwired: 6 in, 3 out]
          }
          frame "ação 3" {
            n192 = local read "Sensor Position 2"() -> (w446:dbl)
            n193 = Greater?(x=w446, y=10.0) -> (0:w447:bool)
            n194 = call <vilib>:"WPI_RobotDriveTankDrive.vi"("Right axis value"=0.5 ("Left axis value"), "Left axis value"=0.5, "RobotDriveDevRef"=w450) -> ()  [unwired: 6 in, 3 out]
            n195 = case shown="True" w447 {
              tunnel: w444 -> [_ w454]
              tunnel: [T2."ação 3" T2."ação 4"] -> w443
              frame False {
              }
              frame True {
                n196 = call <vilib>:"SPARK Set Sensor Position.vi"("Position"=0.0, "MotorControlDeviceRef"=w454) -> ()  [unwired: 8 in, 2 out]
              }
            }
          }
          frame "ação 4" {
            n197 = local read "Sensor Position 2"() -> (w460:dbl)
            n198 = call <vilib>:"WPI_RobotDriveTankDrive.vi"("Right axis value"=-0.5 ("Left axis value"), "Left axis value"=0.5, "RobotDriveDevRef"=w463) -> ()  [unwired: 6 in, 3 out]
            n199 = Less?(x=w460, y=-10.0) -> (x < y?=w458:bool)
            n200 = case shown="True" w458 {
              tunnel: w457 -> [_ w467]
              tunnel: [T2."ação 4" T2."ação 5"] -> w456
              frame False {
              }
              frame True {
                n201 = call <vilib>:"SPARK Set Sensor Position.vi"("Position"=0.0, "MotorControlDeviceRef"=w467) -> ()  [unwired: 8 in, 2 out]
              }
            }
          }
          frame "ação 5" {
            n202 = local read "Sensor Position 2"() -> (w472:dbl)
            n203 = call <vilib>:"WPI_RobotDriveTankDrive.vi"("Right axis value"=-0.5 ("Left axis value"), "Left axis value"=-0.5, "RobotDriveDevRef"=w473) -> ()  [unwired: 6 in, 3 out]
            n204 = Less?(x=w472, y=-13.0) -> (x < y?=w470:bool)
            n205 = case shown="True" w470 {
              tunnel: w476 -> [_ w479]
              tunnel: [T2."ação 5" T2."ação 7"] -> w469
              frame False {
              }
              frame True {
                n206 = call <vilib>:"SPARK Set Sensor Position.vi"("Position"=0.0, "MotorControlDeviceRef"=w479) -> ()  [unwired: 8 in, 2 out]
              }
            }
          }
          frame "ação 7" {
            n207 = local read "Sensor Position 2"() -> (w486:dbl)
            n208 = call <vilib>:"WPI_RobotDriveTankDrive.vi"("Right axis value"=-0.5 ("Left axis value"), "Left axis value"=0.5, "RobotDriveDevRef"=w489) -> ()  [unwired: 6 in, 3 out]
            n209 = Less?(x=w486, y=-10.0) -> (x < y?=w484:bool)
            n210 = case shown="True" w484 {
              tunnel: w483 -> [_ w493]
              tunnel: [T2."ação 7" T2."ação 8"] -> w482
              frame False {
              }
              frame True {
                n211 = call <vilib>:"SPARK Set Sensor Position.vi"("Position"=0.0, "MotorControlDeviceRef"=w493) -> ()  [unwired: 8 in, 2 out]
              }
            }
          }
          frame "ação 8" {
            n212 = local read "Sensor Position 2"() -> (w498:dbl)
            n213 = call <vilib>:"WPI_RobotDriveTankDrive.vi"("Right axis value"=-0.5 ("Left axis value"), "Left axis value"=-0.5, "RobotDriveDevRef"=w501) -> ("RobotDriveDevRef"=w496:T5)  [unwired: 6 in, 2 out]
            n214 = Less?(x=w498, y=-100.0) -> (x < y?=w495:bool)
            n215 = case shown="True" w495 {
              tunnel: w496 -> [_ w504]
              frame False {
              }
              frame True {
                n216 = call <vilib>:"WPI_RobotDriveTankDrive.vi"("Right axis value"=0.0 ("Left axis value"), "Left axis value"=0.0, "RobotDriveDevRef"=w504) -> ()  [unwired: 6 in, 3 out]
              }
            }
          }
        }
        n217 = Wait (ms)(milliseconds to wait=u32 20) -> ()  [unwired: 1 out]
      }
    }
    frame "meio ld azul" {
      n218 = call <vilib>:"WPI_RobotDriveRefNum Registry Get.vi"("refnum name"="tracao") -> ("error out"=w524:errorcluster, "RobotDriveDevRef"=w523:T5)  [unwired: 9 in]
      n219 = call <vilib>:"WPI_RobotDriveRefNum Registry Get.vi"("refnum name"="rd") -> ("RobotDriveDevRef"=w513:T5)  [unwired: 9 in, 1 out]
      n220 = call <vilib>:"WPI_RobotDriveSafetyConfig.vi"("error in (no error)"=w524, "mode"=WPI_SafetyOutputConfigMenu."Enable", "RobotDriveDevRef"=w523) -> ("RobotDriveDevRef"=w511:T5)  [unwired: 7 in, 1 out]
      n221 = call <vilib>:"WPI_RobotDriveSafetyConfig.vi"("mode"=WPI_SafetyOutputConfigMenu."Enable", "RobotDriveDevRef"=w513) -> ("RobotDriveDevRef"=w512:T5)  [unwired: 8 in, 1 out]
      n222 = Unbundle By Name(w511) -> ("Motors[]"=w522:T6[])
      n223 = Index Array(array=w522) -> (element #1=w515:T6, element #2=w519:T6, element #3=w518:T6, element #4=w517:T6)  [unwired: 4 in]
      n224 = call <vilib>:"SPARK Set Idle Mode.vi"("Idle Mode"=Spark_MAX_Idle_Mode."Brake", "MotorControlDeviceRef in"=w515) -> ()  [unwired: 8 in, 2 out]
      n225 = call <vilib>:"SPARK Set Idle Mode.vi"("Idle Mode"=Spark_MAX_Idle_Mode."Brake", "MotorControlDeviceRef in"=w519) -> ()  [unwired: 8 in, 2 out]
      n226 = call <vilib>:"SPARK Set Idle Mode.vi"("Idle Mode"=Spark_MAX_Idle_Mode."Brake", "MotorControlDeviceRef in"=w518) -> ()  [unwired: 8 in, 2 out]
      n227 = call <vilib>:"SPARK Set Idle Mode.vi"("Idle Mode"=Spark_MAX_Idle_Mode."Brake", "MotorControlDeviceRef in"=w517) -> ()  [unwired: 8 in, 2 out]
      n228 = call <vilib>:"SPARK Set Sensor Position.vi"("Position"=0.0, "MotorControlDeviceRef"=w515) -> ("MotorControlDeviceRef"=w510:T6)  [unwired: 8 in, 1 out]
      n229 = while {
        shift-right: [w531] -> _
        shift-left: T2."ação 8" -> [w533]
        tunnel: w512 -> [w532]
        tunnel: w511 -> [w530]
        tunnel: w510 -> [w528]
        stop <- w526 stop-if-true
        n230 = call <vilib>:"SPARK Get Sensor Position.vi"("MotorControlDevRef in"=w528) -> ("Sensor Position"=→"Sensor Position 5":dbl, "MotorControlDevRef out"=w527:T6)  [unwired: 7 in, 2 out]
        n231 = case shown="\"ação 7\"" w533 {
          tunnel: w532 -> [w541 w553 _ _ _ _ _]
          tunnel: [w536 T2."ação 3" w555 w568 w581 w594 T2."ação 8"] -> w531
          tunnel: w530 -> [_ _ w562 w575 w585 w601 w613]
          tunnel: w527 -> [_ _ w556 w569 w588 w595 _]
          tunnel: [FALSE FALSE FALSE FALSE FALSE FALSE w607] -> w526
          frame "ação 1", Default {
            n232 = Tick Count (ms)() -> (millisecond timer value=w539:u32)
            n233 = call <vilib>:"WPI_RobotDriveTankDrive.vi"("Right axis value"=1.0, "Left axis value"=0.0, "RobotDriveDevRef"=w541) -> ("RobotDriveDevRef"=w540:T5)  [unwired: 6 in, 2 out]
            n234 = Greater?(x=w539, y=u32 1000) -> (0:w537:bool)
            n235 = case shown="True" w537 {
              tunnel: w540 -> [_ w546]
              tunnel: [T2."ação 1" T2."ação 2"] -> w536
              frame False {
              }
              frame True {
                n236 = call <vilib>:"WPI_RobotDriveTankDrive.vi"("Right axis value"=1.0 ("Left axis value"), "Left axis value"=1.0 ("Right axis value"), "RobotDriveDevRef"=w546) -> ()  [unwired: 6 in, 3 out]
              }
            }
          }
          frame "ação 2" {
            n237 = call <vilib>:"WPI_RobotDriveTankDrive.vi"("Right axis value"=0.0, "Left axis value"=0.0, "RobotDriveDevRef"=w553) -> ()  [unwired: 6 in, 3 out]
          }
          frame "ação 3" {
            n238 = local read "Sensor Position 5"() -> (w558:dbl)
            n239 = Greater?(x=w558, y=10.0) -> (0:w559:bool)
            n240 = call <vilib>:"WPI_RobotDriveTankDrive.vi"("Right axis value"=0.5 ("Left axis value"), "Left axis value"=0.5, "RobotDriveDevRef"=w562) -> ()  [unwired: 6 in, 3 out]
            n241 = case shown="True" w559 {
              tunnel: w556 -> [_ w566]
              tunnel: [T2."ação 3" T2."ação 4"] -> w555
              frame False {
              }
              frame True {
                n242 = call <vilib>:"SPARK Set Sensor Position.vi"("Position"=0.0, "MotorControlDeviceRef"=w566) -> ()  [unwired: 8 in, 2 out]
              }
            }
          }
          frame "ação 4" {
            n243 = local read "Sensor Position 5"() -> (w572:dbl)
            n244 = call <vilib>:"WPI_RobotDriveTankDrive.vi"("Right axis value"=0.5 ("Left axis value"), "Left axis value"=-0.5, "RobotDriveDevRef"=w575) -> ()  [unwired: 6 in, 3 out]
            n245 = Greater?(x=w572, y=10.0) -> (0:w570:bool)
            n246 = case shown="True" w570 {
              tunnel: w569 -> [_ w579]
              tunnel: [T2."ação 4" T2."ação 5"] -> w568
              frame False {
              }
              frame True {
                n247 = call <vilib>:"SPARK Set Sensor Position.vi"("Position"=0.0, "MotorControlDeviceRef"=w579) -> ()  [unwired: 8 in, 2 out]
              }
            }
          }
          frame "ação 5" {
            n248 = local read "Sensor Position 5"() -> (w584:dbl)
            n249 = call <vilib>:"WPI_RobotDriveTankDrive.vi"("Right axis value"=-0.5 ("Left axis value"), "Left axis value"=-0.5, "RobotDriveDevRef"=w585) -> ()  [unwired: 6 in, 3 out]
            n250 = Less?(x=w584, y=-13.0) -> (x < y?=w582:bool)
            n251 = case shown="True" w582 {
              tunnel: w588 -> [_ w591]
              tunnel: [T2."ação 5" T2."ação 7"] -> w581
              frame False {
              }
              frame True {
                n252 = call <vilib>:"SPARK Set Sensor Position.vi"("Position"=0.0, "MotorControlDeviceRef"=w591) -> ()  [unwired: 8 in, 2 out]
              }
            }
          }
          frame "ação 7" {
            n253 = local read "Sensor Position 5"() -> (w598:dbl)
            n254 = call <vilib>:"WPI_RobotDriveTankDrive.vi"("Right axis value"=0.5 ("Left axis value"), "Left axis value"=-0.5, "RobotDriveDevRef"=w601) -> ()  [unwired: 6 in, 3 out]
            n255 = Greater?(x=w598, y=10.0) -> (0:w596:bool)
            n256 = case shown="True" w596 {
              tunnel: w595 -> [_ w605]
              tunnel: [T2."ação 7" T2."ação 8"] -> w594
              frame False {
              }
              frame True {
                n257 = call <vilib>:"SPARK Set Sensor Position.vi"("Position"=0.0, "MotorControlDeviceRef"=w605) -> ()  [unwired: 8 in, 2 out]
              }
            }
          }
          frame "ação 8" {
            n258 = local read "Sensor Position 5"() -> (w610:dbl)
            n259 = call <vilib>:"WPI_RobotDriveTankDrive.vi"("Right axis value"=-0.5 ("Left axis value"), "Left axis value"=-0.5, "RobotDriveDevRef"=w613) -> ("RobotDriveDevRef"=w608:T5)  [unwired: 6 in, 2 out]
            n260 = Less?(x=w610, y=-100.0) -> (x < y?=w607:bool)
            n261 = case shown="True" w607 {
              tunnel: w608 -> [_ w616]
              frame False {
              }
              frame True {
                n262 = call <vilib>:"WPI_RobotDriveTankDrive.vi"("Right axis value"=0.0 ("Left axis value"), "Left axis value"=0.0, "RobotDriveDevRef"=w616) -> ()  [unwired: 6 in, 3 out]
              }
            }
          }
        }
        n263 = Wait (ms)(milliseconds to wait=u32 20) -> ()  [unwired: 1 out]
      }
    }
    frame "esquerda" {
      n264 = call <vilib>:"WPI_RobotDriveRefNum Registry Get.vi"("refnum name"="rd") -> ("RobotDriveDevRef"=w626:T5)  [unwired: 9 in, 1 out]
      n265 = call <vilib>:"WPI_RobotDriveRefNum Registry Get.vi"("refnum name"="tracao") -> ("error out"=w636:errorcluster, "RobotDriveDevRef"=w635:T5)  [unwired: 9 in]
      n266 = call <vilib>:"WPI_RobotDriveSafetyConfig.vi"("error in (no error)"=w636, "mode"=WPI_SafetyOutputConfigMenu."Enable", "RobotDriveDevRef"=w635) -> ("RobotDriveDevRef"=w624:T5)  [unwired: 7 in, 1 out]
      n267 = call <vilib>:"WPI_RobotDriveSafetyConfig.vi"("mode"=WPI_SafetyOutputConfigMenu."Enable", "RobotDriveDevRef"=w626) -> ("RobotDriveDevRef"=w625:T5)  [unwired: 8 in, 1 out]
      n268 = Unbundle By Name(w624) -> ("Motors[]"=w634:T6[])
      n269 = Index Array(array=w634) -> (element #1=w628:T6, element #2=w632:T6, element #3=w631:T6, element #4=w630:T6)  [unwired: 4 in]
      n270 = call <vilib>:"SPARK Set Idle Mode.vi"("Idle Mode"=Spark_MAX_Idle_Mode."Brake", "MotorControlDeviceRef in"=w628) -> ()  [unwired: 8 in, 2 out]
      n271 = call <vilib>:"SPARK Set Idle Mode.vi"("Idle Mode"=Spark_MAX_Idle_Mode."Brake", "MotorControlDeviceRef in"=w632) -> ()  [unwired: 8 in, 2 out]
      n272 = call <vilib>:"SPARK Set Idle Mode.vi"("Idle Mode"=Spark_MAX_Idle_Mode."Brake", "MotorControlDeviceRef in"=w631) -> ()  [unwired: 8 in, 2 out]
      n273 = call <vilib>:"SPARK Set Idle Mode.vi"("Idle Mode"=Spark_MAX_Idle_Mode."Brake", "MotorControlDeviceRef in"=w630) -> ()  [unwired: 8 in, 2 out]
      n274 = call <vilib>:"SPARK Set Sensor Position.vi"("Position"=0.0, "MotorControlDeviceRef"=w628) -> ("MotorControlDeviceRef"=w623:T6)  [unwired: 8 in, 1 out]
      n275 = while {
        shift-right: [w638] -> _
        shift-left: T4."ação 1" -> [w639]
        tunnel: w625 -> [w645]
        tunnel: w624 -> [w644]
        tunnel: w623 -> [w642]
        stop <- w640 stop-if-true
        n276 = call <vilib>:"SPARK Get Sensor Position.vi"("MotorControlDevRef in"=w642) -> ("Sensor Position"=→"Sensor Position 3":dbl, "MotorControlDevRef out"=w641:T6)  [unwired: 7 in, 2 out]
        n277 = case shown="\"ação 4\"" w639 {
          tunnel: w645 -> [w653 w665 _ _ _]
          tunnel: w644 -> [_ _ w674 w687 w697]
          tunnel: w641 -> [_ _ w668 w681 _]
          tunnel: [FALSE FALSE FALSE FALSE w692] -> w640
          tunnel: [w647 T4."ação 3" w666 w679 T4."ação 5"] -> w638
          frame "ação 1", Default {
            n278 = Tick Count (ms)() -> (millisecond timer value=w651:u32)
            n279 = call <vilib>:"WPI_RobotDriveTankDrive.vi"("Right axis value"=1.0, "Left axis value"=0.0, "RobotDriveDevRef"=w653) -> ("RobotDriveDevRef"=w652:T5)  [unwired: 6 in, 2 out]
            n280 = Greater?(x=w651, y=u32 1000) -> (0:w649:bool)
            n281 = case shown="True" w649 {
              tunnel: w652 -> [_ w658]
              tunnel: [T4."ação 1" T4."ação 2"] -> w647
              frame False {
              }
              frame True {
                n282 = call <vilib>:"WPI_RobotDriveTankDrive.vi"("Right axis value"=1.0 ("Left axis value"), "Left axis value"=1.0 ("Right axis value"), "RobotDriveDevRef"=w658) -> ()  [unwired: 6 in, 3 out]
              }
            }
          }
          frame "ação 2" {
            n283 = call <vilib>:"WPI_RobotDriveTankDrive.vi"("Right axis value"=0.0, "Left axis value"=0.0, "RobotDriveDevRef"=w665) -> ()  [unwired: 6 in, 3 out]
          }
          frame "ação 3" {
            n284 = local read "Sensor Position 3"() -> (w670:dbl)
            n285 = Greater?(x=w670, y=57.0) -> (0:w671:bool)
            n286 = call <vilib>:"WPI_RobotDriveTankDrive.vi"("Right axis value"=0.5 ("Left axis value"), "Left axis value"=0.5, "RobotDriveDevRef"=w674) -> ()  [unwired: 6 in, 3 out]
            n287 = case shown="False" w671 {
              tunnel: w668 -> [_ w678]
              tunnel: [T4."ação 3" T4."ação 4"] -> w666
              frame False {
              }
              frame True {
                n288 = call <vilib>:"SPARK Set Sensor Position.vi"("Position"=0.0, "MotorControlDeviceRef"=w678) -> ()  [unwired: 8 in, 2 out]
              }
            }
          }
          frame "ação 4" {
            n289 = local read "Sensor Position 3"() -> (w684:dbl)
            n290 = call <vilib>:"WPI_RobotDriveTankDrive.vi"("Right axis value"=-0.5 ("Left axis value"), "Left axis value"=0.5, "RobotDriveDevRef"=w687) -> ()  [unwired: 6 in, 3 out]
            n291 = Less?(x=w684, y=-10.0) -> (x < y?=w682:bool)
            n292 = case shown="False" w682 {
              tunnel: w681 -> [_ w691]
              tunnel: [T4."ação 4" T4."ação 5"] -> w679
              frame False {
              }
              frame True {
                n293 = call <vilib>:"SPARK Set Sensor Position.vi"("Position"=0.0, "MotorControlDeviceRef"=w691) -> ()  [unwired: 8 in, 2 out]
              }
            }
          }
          frame "ação 5" {
            n294 = local read "Sensor Position 3"() -> (w696:dbl)
            n295 = call <vilib>:"WPI_RobotDriveTankDrive.vi"("Right axis value"=-0.5 ("Left axis value"), "Left axis value"=-0.5, "RobotDriveDevRef"=w697) -> ("RobotDriveDevRef"=w694:T5)  [unwired: 6 in, 2 out]
            n296 = Less?(x=w696, y=-60.0) -> (x < y?=w692:bool)
            n297 = case shown="False" w692 {
              tunnel: w694 -> [_ w700]
              frame False {
              }
              frame True {
                n298 = call <vilib>:"WPI_RobotDriveTankDrive.vi"("Right axis value"=0.0 ("Left axis value"), "Left axis value"=0.0, "RobotDriveDevRef"=w700) -> ()  [unwired: 6 in, 3 out]
              }
            }
          }
        }
        n299 = Wait (ms)(milliseconds to wait=u32 20) -> ()  [unwired: 1 out]
      }
    }
    frame "esquerda azul" {
      n300 = call <vilib>:"WPI_RobotDriveRefNum Registry Get.vi"("refnum name"="rd") -> ("RobotDriveDevRef"=w712:T5)  [unwired: 9 in, 1 out]
      n301 = call <vilib>:"WPI_RobotDriveRefNum Registry Get.vi"("refnum name"="tracao") -> ("error out"=w722:errorcluster, "RobotDriveDevRef"=w721:T5)  [unwired: 9 in]
      n302 = call <vilib>:"WPI_RobotDriveSafetyConfig.vi"("error in (no error)"=w722, "mode"=WPI_SafetyOutputConfigMenu."Enable", "RobotDriveDevRef"=w721) -> ("RobotDriveDevRef"=w710:T5)  [unwired: 7 in, 1 out]
      n303 = call <vilib>:"WPI_RobotDriveSafetyConfig.vi"("mode"=WPI_SafetyOutputConfigMenu."Enable", "RobotDriveDevRef"=w712) -> ("RobotDriveDevRef"=w711:T5)  [unwired: 8 in, 1 out]
      n304 = Unbundle By Name(w710) -> ("Motors[]"=w720:T6[])
      n305 = Index Array(array=w720) -> (element #1=w714:T6, element #2=w718:T6, element #3=w717:T6, element #4=w716:T6)  [unwired: 4 in]
      n306 = call <vilib>:"SPARK Set Idle Mode.vi"("Idle Mode"=Spark_MAX_Idle_Mode."Brake", "MotorControlDeviceRef in"=w714) -> ()  [unwired: 8 in, 2 out]
      n307 = call <vilib>:"SPARK Set Idle Mode.vi"("Idle Mode"=Spark_MAX_Idle_Mode."Brake", "MotorControlDeviceRef in"=w718) -> ()  [unwired: 8 in, 2 out]
      n308 = call <vilib>:"SPARK Set Idle Mode.vi"("Idle Mode"=Spark_MAX_Idle_Mode."Brake", "MotorControlDeviceRef in"=w717) -> ()  [unwired: 8 in, 2 out]
      n309 = call <vilib>:"SPARK Set Idle Mode.vi"("Idle Mode"=Spark_MAX_Idle_Mode."Brake", "MotorControlDeviceRef in"=w716) -> ()  [unwired: 8 in, 2 out]
      n310 = call <vilib>:"SPARK Set Sensor Position.vi"("Position"=0.0, "MotorControlDeviceRef"=w714) -> ("MotorControlDeviceRef"=w709:T6)  [unwired: 8 in, 1 out]
      n311 = while {
        shift-right: [w724] -> _
        shift-left: T4."ação 1" -> [w725]
        tunnel: w711 -> [w731]
        tunnel: w710 -> [w730]
        tunnel: w709 -> [w728]
        stop <- w726 stop-if-true
        n312 = call <vilib>:"SPARK Get Sensor Position.vi"("MotorControlDevRef in"=w728) -> ("Sensor Position"=→"Sensor Position 4":dbl, "MotorControlDevRef out"=w727:T6)  [unwired: 7 in, 2 out]
        n313 = case shown="\"ação 1\", Default" w725 {
          tunnel: w731 -> [w739 w751 _ _ _]
          tunnel: w730 -> [_ _ w760 w773 w783]
          tunnel: w727 -> [_ _ w754 w767 _]
          tunnel: [FALSE FALSE FALSE FALSE w778] -> w726
          tunnel: [w733 T4."ação 3" w752 w765 T4."ação 5"] -> w724
          frame "ação 1", Default {
            n314 = Tick Count (ms)() -> (millisecond timer value=w737:u32)
            n315 = call <vilib>:"WPI_RobotDriveTankDrive.vi"("Right axis value"=1.0, "Left axis value"=0.0, "RobotDriveDevRef"=w739) -> ("RobotDriveDevRef"=w738:T5)  [unwired: 6 in, 2 out]
            n316 = Greater?(x=w737, y=u32 1000) -> (0:w735:bool)
            n317 = case shown="True" w735 {
              tunnel: w738 -> [_ w744]
              tunnel: [T4."ação 1" T4."ação 2"] -> w733
              frame False {
              }
              frame True {
                n318 = call <vilib>:"WPI_RobotDriveTankDrive.vi"("Right axis value"=1.0 ("Left axis value"), "Left axis value"=1.0 ("Right axis value"), "RobotDriveDevRef"=w744) -> ()  [unwired: 6 in, 3 out]
              }
            }
          }
          frame "ação 2" {
            n319 = call <vilib>:"WPI_RobotDriveTankDrive.vi"("Right axis value"=0.0, "Left axis value"=0.0, "RobotDriveDevRef"=w751) -> ()  [unwired: 6 in, 3 out]
          }
          frame "ação 3" {
            n320 = local read "Sensor Position 4"() -> (w756:dbl)
            n321 = Greater?(x=w756, y=57.0) -> (0:w757:bool)
            n322 = call <vilib>:"WPI_RobotDriveTankDrive.vi"("Right axis value"=0.5 ("Left axis value"), "Left axis value"=0.5, "RobotDriveDevRef"=w760) -> ()  [unwired: 6 in, 3 out]
            n323 = case shown="False" w757 {
              tunnel: w754 -> [_ w764]
              tunnel: [T4."ação 3" T4."ação 4"] -> w752
              frame False {
              }
              frame True {
                n324 = call <vilib>:"SPARK Set Sensor Position.vi"("Position"=0.0, "MotorControlDeviceRef"=w764) -> ()  [unwired: 8 in, 2 out]
              }
            }
          }
          frame "ação 4" {
            n325 = local read "Sensor Position 4"() -> (w770:dbl)
            n326 = call <vilib>:"WPI_RobotDriveTankDrive.vi"("Right axis value"=0.5 ("Left axis value"), "Left axis value"=-0.5, "RobotDriveDevRef"=w773) -> ()  [unwired: 6 in, 3 out]
            n327 = Greater?(x=w770, y=10.0) -> (0:w768:bool)
            n328 = case shown="False" w768 {
              tunnel: w767 -> [_ w777]
              tunnel: [T4."ação 4" T4."ação 5"] -> w765
              frame False {
              }
              frame True {
                n329 = call <vilib>:"SPARK Set Sensor Position.vi"("Position"=0.0, "MotorControlDeviceRef"=w777) -> ()  [unwired: 8 in, 2 out]
              }
            }
          }
          frame "ação 5" {
            n330 = local read "Sensor Position 4"() -> (w782:dbl)
            n331 = call <vilib>:"WPI_RobotDriveTankDrive.vi"("Right axis value"=-0.5 ("Left axis value"), "Left axis value"=-0.5, "RobotDriveDevRef"=w783) -> ("RobotDriveDevRef"=w780:T5)  [unwired: 6 in, 2 out]
            n332 = Less?(x=w782, y=-60.0) -> (x < y?=w778:bool)
            n333 = case shown="False" w778 {
              tunnel: w780 -> [_ w786]
              frame False {
              }
              frame True {
                n334 = call <vilib>:"WPI_RobotDriveTankDrive.vi"("Right axis value"=0.0 ("Left axis value"), "Left axis value"=0.0, "RobotDriveDevRef"=w786) -> ()  [unwired: 6 in, 3 out]
              }
            }
          }
        }
        n335 = Wait (ms)(milliseconds to wait=u32 20) -> ()  [unwired: 1 out]
      }
    }
    frame "teste shooter" {
      n336 = call <vilib>:"WPI_RobotDriveRefNum Registry Get.vi"("refnum name"="rd") -> ("RobotDriveDevRef"=w794:T5)  [unwired: 9 in, 1 out]
      n337 = call <vilib>:"WPI_RobotDriveTankDrive.vi"("Right axis value"=1.0 ("Left axis value"), "Left axis value"=1.0, "RobotDriveDevRef"=w794) -> ("RobotDriveDevRef"=w789:T5)  [unwired: 6 in, 2 out]
      n338 = Unbundle By Name(w789) -> ("Motors[]"=w790:T6[])
      n339 = while {
        tunnel: w790 -> [w802]
        stop <- w799 stop-if-true
        n340 = Index Array(array=w802) -> (element #1=w807:T6, element #2=w806:T6)  [unwired: 2 in]
        n341 = Wait (ms)(milliseconds to wait=u32 20) -> ()  [unwired: 1 out]
        n342 = call <vilib>:"SPARK Get Sensor Position.vi"("MotorControlDevRef in"=w806) -> ("Sensor Position"=w805:dbl, "MotorControlDevRef out"=w797:T6)  [unwired: 7 in, 2 out]
        "Sensor Position 7" <- w805
        n343 = call <vilib>:"SPARK Get Sensor Position.vi"("MotorControlDevRef in"=w807) -> ("Sensor Position"=w795:dbl, "MotorControlDevRef out"=w796:T6)  [unwired: 7 in, 2 out]
        "Sensor Position 8" <- w795
        n344 = Greater?(x=w805, y=50.0) -> (0:w800:bool)
        n345 = Greater?(x=w795, y=50.0) -> (0:w801:bool)
        n346 = And(x=w801, y=w800) -> (x .and. y?=w799:bool)
        n347 = case shown="True" w801 {
          tunnel: w796 -> [_ w815]
          frame False {
          }
          frame True {
            n348 = call <vilib>:"WPI_MotorControlSetOutput.vi"("Output"=0.0, "MotorControlDevRef"=w815) -> ("MotorControlDevRef"=w813:T6)  [unwired: 7 in, 2 out]
            n349 = call <vilib>:"SPARK Set Sensor Position.vi"("Position"=0.0, "MotorControlDeviceRef"=w813) -> ()  [unwired: 8 in, 2 out]
          }
        }
        n350 = case shown="True" w800 {
          tunnel: w797 -> [_ w811]
          frame False {
          }
          frame True {
            n351 = call <vilib>:"WPI_MotorControlSetOutput.vi"("Output"=0.0, "MotorControlDevRef"=w811) -> ("MotorControlDevRef"=w809:T6)  [unwired: 7 in, 2 out]
            n352 = call <vilib>:"SPARK Set Sensor Position.vi"("Position"=0.0, "MotorControlDeviceRef"=w809) -> ()  [unwired: 8 in, 2 out]
          }
        }
      }
    }
  }
